vi "Build Image File Names.vi"(8 "error in (no error)":errorcluster, 11 "Controller in":refnum<class "Controller.lvclass">) -> (0 "error out":errorcluster, 2 "Paths":path[](array[path]), 3 "Controller out":refnum<class "Controller.lvclass">)   [LabVIEW 2022 SP3, in "Controller.lvlib" / "Controller.lvclass"]
uses:
  Controller.lvclass
  Controller.lvclass/Controller.ctl
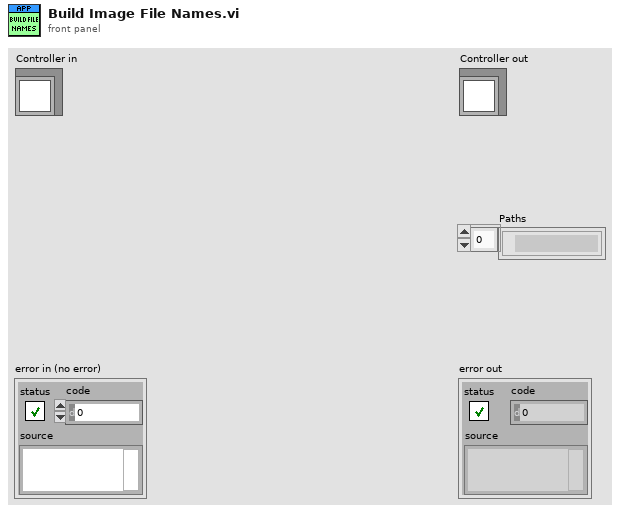
[diagram p1: front panel]
types:
  T1 = typedef "Image Formats.ctl" = enum16{"<Select>", "TIFF", "RAW"}
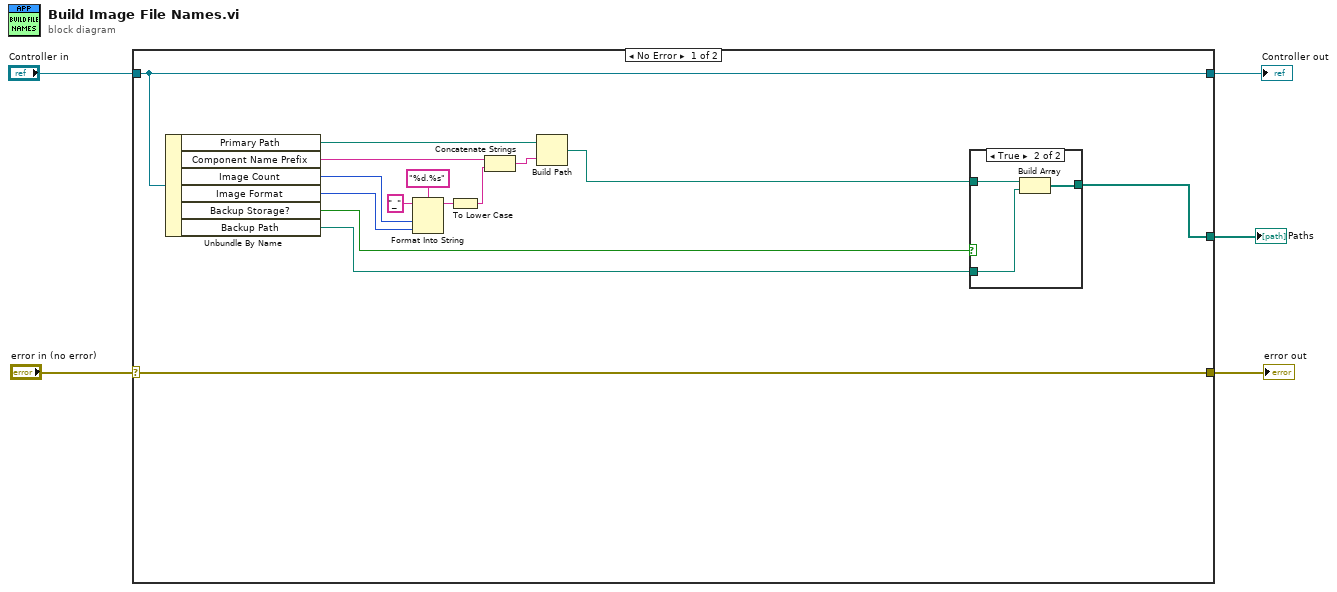
[diagram p0: block diagram]
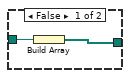
[diagram p2: hidden frame]
diagram:
  n1 = case shown="No Error" "error in (no error)" {
    selector: "error in (no error)" -> [w20 w27]
    tunnel: [w20 w27] -> w4
    tunnel: [w19 w26] -> w2
    tunnel: "Controller in" -> [w19 w26]
    tunnel: [w7 _] -> w1
    frame No Error {
      n2 = Unbundle By Name(w19) -> ("Primary Path"=w6:path, "Component Name Prefix"=w16:string, "Image Count"=w14:u32, "Image Format"=w13:T1, "Backup Storage?"=w10:bool, "Backup Path"=w9:path)
      n3 = Format Into String(format string="%d.%s", initial string="_", w14, w13) -> (resulting string=w18:string)  [unwired: 1 in, 1 out]
      n4 = To Lower Case(string=w18) -> (all lower case string=w17:string)
      n5 = Concatenate Strings(w16, w17) -> (w11:string)
      n6 = Build Path(base path=w6, name or relative path=w11) -> (appended path=w8:path)
      n7 = case shown="True" w10 {
        tunnel: w9 -> [_ w24]
        tunnel: w8 -> [w22 w25]
        tunnel: [w21 w23] -> w7
        frame False {
          n8 = Build Array(w22) -> (w21:path[])
        }
        frame True {
          n9 = Build Array(w25, w24) -> (w23:path[])
        }
      }
    }
    frame Error {
    }
  }
  "error out" <- w4
  "Controller out" <- w2
  "Paths" <- w1
